vi "Write Error.vi"(8 "error in (no error)":errorcluster, 10 "error":errorcluster, 11 "GET Async in":refnum<class "GET Async.lvclass">) -> (0 "error out":errorcluster, 3 "GET Async out":refnum<class "GET Async.lvclass">)   [LabVIEW 2019, in "HTTP Client Extensions.lvlib" / "GET Async.lvclass"]
uses:
  GET Async.lvclass
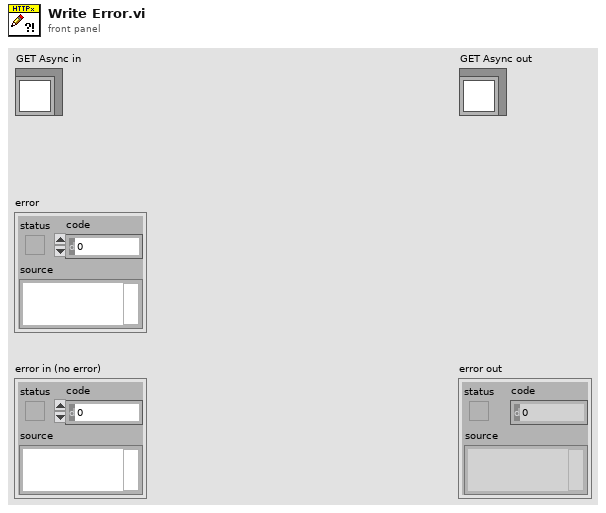
[diagram p1: front panel]
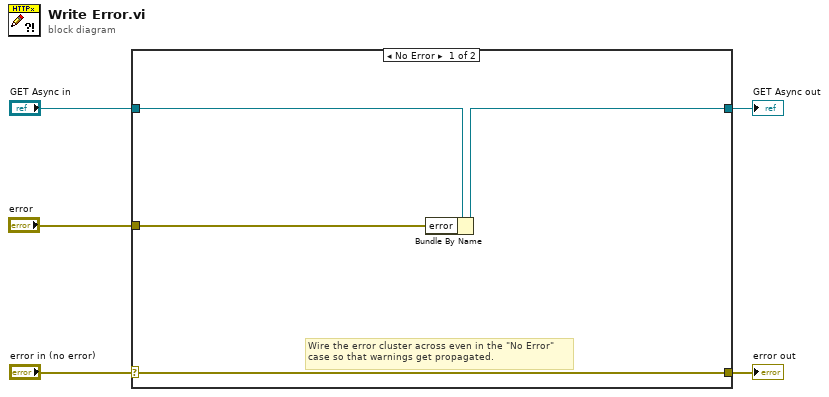
[diagram p0: block diagram]
diagram:
  n1 = case shown="No Error" "error in (no error)" {
    selector: "error in (no error)" -> [w8 w11]
    tunnel: [w8 w11] -> w4
    tunnel: [w7 w10] -> w2
    tunnel: "GET Async in" -> [w9 w10]
    tunnel: "error" -> [w6 _]
    frame No Error {
      # "Wire the error cluster across even in the \"No Error\"\ncase so that warnings get propagated."
      n2 = Bundle By Name(cluster=w9, "error"=w6) -> (w7:refnum<class "GET Async.lvclass">)
    }
    frame Error {
    }
  }
  "error out" <- w4
  "GET Async out" <- w2
